vi "from string.vi"(8 "error in":errorcluster, 9 "data":string, 10 "version":string, 11 "Submodule EOL configuration":refnum<class "Submodule EOL configuration.lvclass">) -> (0 "error out":errorcluster, 3 "Submodule EOL configuration out":refnum<class "Submodule EOL configuration.lvclass">)   [LabVIEW 2025, in "Submodule EOL.lvlib" / "Submodule EOL configuration.lvclass"]
doc: "Provides an interface for loading a module configuration from a file or other serialized data source. It is recommended that all children of this class store data in two sets--data required for its own initialization, and any data required for parent initialization--and that each implementation uses the <b>Call Parent Method</b> primitive to de-serialize parent information.Copyright 2017 National Instruments Corporation\n\nLicensed under the Apache License, Version 2.0 (the \"License\"); you may not use this file except in compliance with the License. You may obtain a copy of the License at http://www.apache.org/licenses/LICENSE-2.0\nUnless required by applicable law or agreed to in writing, software distributed under the License is distributed on an \"AS IS\" BASIS, WITHOUT WARRANTIES OR CONDITIONS OF ANY KIND, either express or implied. See the License for the specific language governing permissions and limitations under the License."
uses:
  Submodule EOL configuration.lvclass
  Submodule EOL configuration.lvclass/Submodule EOL configuration.ctl
  Users/Public/Documents/Sandia National Labs/TSS Plugin/CEF.lvlibp/serializable configuration/CEF_serializable configuration.lvclass
  Submodule EOL.ctl
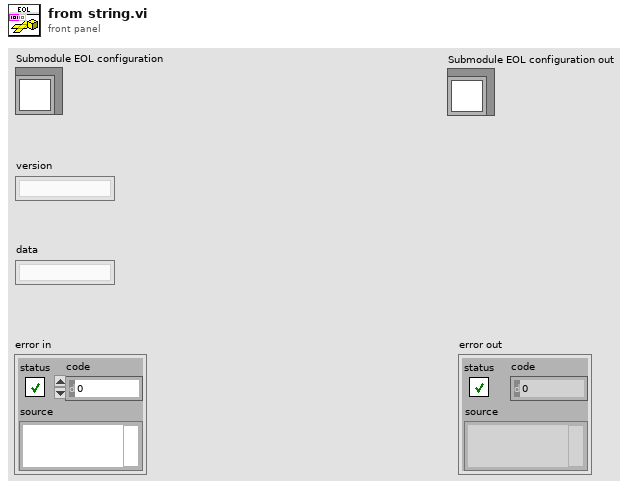
[diagram p1: front panel]
types:
  T1 = typedef "Submodule EOL.lvlib/Submodule EOL configuration.lvclass/Submodule EOL.ctl" = cluster{"PLC Folder Names":string[][], "Timeout Connect OPC":dbl, "Connect OPC Trial":u32, "PLC URL":string, "Digitial IO":string, "HiPOT":string, "ACIR with Switch":string, "DMM with Switch":string, "Ignition Folder Names":string[][], "Ignition URL":string}
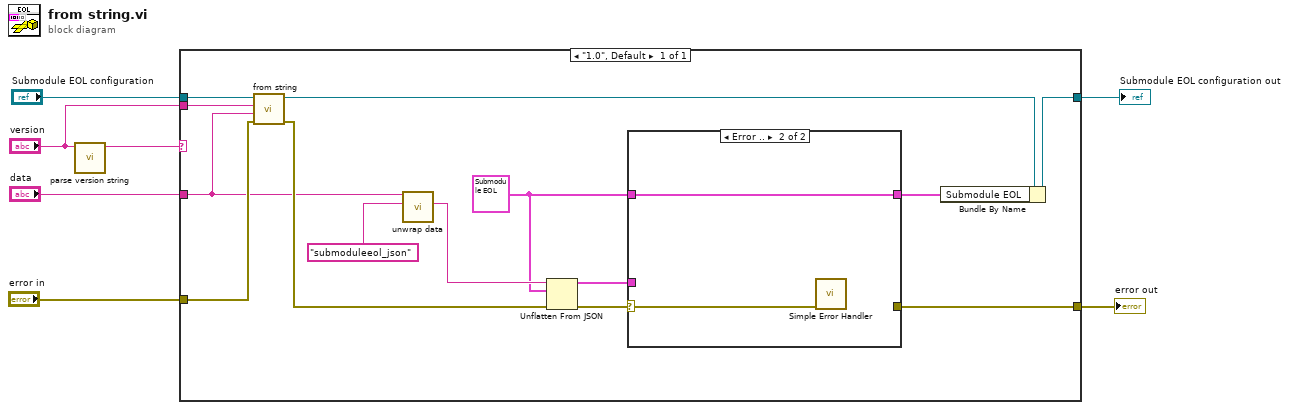
[diagram p0: block diagram]
diagram:
  n1 = call "parse version string.vi"("full version"="version") -> ("major.minor version"=w5:string)  [unwired: 7 in, 3 out]
  n2 = case shown="\"1.0\", Default" w5 {
    tunnel: "Submodule EOL configuration" -> [w21]
    tunnel: [w17] -> w1
    tunnel: "data" -> [w13]
    tunnel: "error in" -> [w19]
    tunnel: [w9] -> w4
    tunnel: "version" -> [w14]
    frame "1.0", Default {
      w11 = T1 {"PLC Folder Names"=[["Station0_Rx", "OP50A_TesterRxSignals"], ["Station0_Tx", "OP50A_TesterTxSignals"], ["Station1_Rx", "OP50B_TesterRxSignals"], ["Station1_Tx", "OP50B_TesterTxSignals"], ["Station2_Rx", "OP60A_TesterRxSignals"], ["Station2_Tx", "OP60A_TesterTxSignals"], ["Station3_Rx", "OP60B_TesterRxSignals"], ["Station3_Tx", "OP60B_TesterTxSignals"], ["Station4_Rx", "OP70A_TesterRxSignals"], ["Station4_Tx", "OP70A_TesterTxSignals"], ["Station5_Rx", "OP70B_TesterRxSignals"], ["Station5_Tx", "OP70B_TesterTxSignals"]], "Timeout Connect OPC"=5.0, "Connect OPC Trial"=3, "PLC URL"="opc.tcp://localhost:49580 ", "Digitial IO"="com0->ch0", "HiPOT"="com0->ch0", "ACIR with Switch"="com0->ch0", "DMM with Switch"="com0->ch0", "Ignition Folder Names"=[["Ignition0_Rx", "[Submodule_EOL]/StaA/TesterRx"], ["Ignition0_Tx", "[Submodule_EOL]/StaA/TesterTx"], ["Ignition1_Rx", "[Submodule_EOL]/StaB/TesterRx"], ["Ignition1_Tx", "[Submodule_EOL]/StaB/TesterTx"], ["Ignition2_Rx", "[Submodule_EOL]/StaC/TesterRx"], ["Ignition2_Tx", "[Submodule_EOL]/StaC/TesterTx"], ["Ignition3_Rx", "[Submodule_EOL]/StaD/TesterRx"], ["Ignition3_Tx", "[Submodule_EOL]/StaD/TesterTx"], ["Ignition4_Rx", "[Submodule_EOL]/StaE/TesterRx"], ["Ignition4_Tx", "[Submodule_EOL]/StaE/TesterTx"], ["Ignition5_Rx", "[Submodule_EOL]/StaF/TesterRx"], ["Ignition5_Tx", "[Submodule_EOL]/StaF/TesterTx"]], "Ignition URL"="opc.tcp://10.64.0.22:62541/discovery"} ("Event")
      n3 = call-parent "from string.vi"("error in"=w19, "data"=w13, "version"=w14, "CEF_Configuration in"=w21) -> ("error out"=w18:errorcluster, "CEF_Configuration out"=w20:refnum<class "Submodule EOL configuration.lvclass">)  [unwired: 6 in]
      n4 = call "unwrap data.vi"("identifier"="submoduleeol_json" ("additional identifier"), "data to unwrap"=w13) -> ("unwrapped data"=w15:string)  [unwired: 8 in, 1 out]
      n5 = Unflatten From JSON(JSON string=w15, type and defaults=w11, error in (no error)=w18) -> (value=w10:T1, error out=w12:errorcluster)  [unwired: 4 in]
      n6 = case shown="Error .." w12 {
        selector: w12 -> [w22 w25]
        tunnel: w10 -> [w23 _]
        tunnel: [w23 w24] -> w8
        tunnel: w11 -> [_ w24]
        tunnel: [w22 _] -> w9
        frame No Error {
        }
        frame Error {
          n7 = call <vilib>:"Simple Error Handler.vi"("error in (no error)"=w25) -> ()  [unwired: 4 in, 5 out]
        }
      }
      n8 = Bundle By Name(cluster=w20, "Submodule EOL"=w8) -> (w17:refnum<class "Submodule EOL configuration.lvclass">)
    }
  }
  "error out" <- w4
  "Submodule EOL configuration out" <- w1
